vi "Color_num_var.vi"() -> ()   [LabVIEW 2019]
panel:
  in  "Color now":dbl
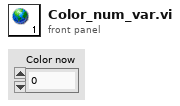
[diagram p1: front panel]
diagram:
